vi "TCPtaskhandle.vi"(6 "心跳包":refnum<vi>, 9 "配置信息":refnum<vi>, 10 "状态信息":refnum<vi>, 11 "通信状态":refnum<vi>) -> ()   [LabVIEW 2016, in "数据传输系统-06.lvlib"]
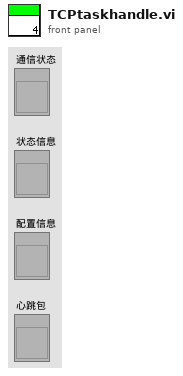
[diagram p1: front panel]
types:
  T1 = cluster{"步骤":enum16{"打开连接", "发送数据", "读取数据", "数据处理", "关闭连接"}, "发送报文":string}
  T2 = cluster{"setini":string, "sysini":string, "hechaini":string, "actualwrite":string, "actualread":string, "datasent":string, "反控命令信息队列":string, "反控与仪器交互":string}
  T3 = cluster{"1st Error to Convert ":i32, "步骤 ":enum16{"打开连接", "发送数据", "读取数据", "数据处理", "关闭连接"}, "元素":string, "TCP服务端掉线计数":i32, "TCP掉线时间节点":string}
  T4 = cluster{"站点":string, "设备":string, "IP":string, "PORT":string, "MN":string, "PW":string}
  T5 = cluster{"枚举":enum16{"打开连接", "发送数据", "读取数据", "数据处理", "关闭连接"}, "读取缓冲区":string}
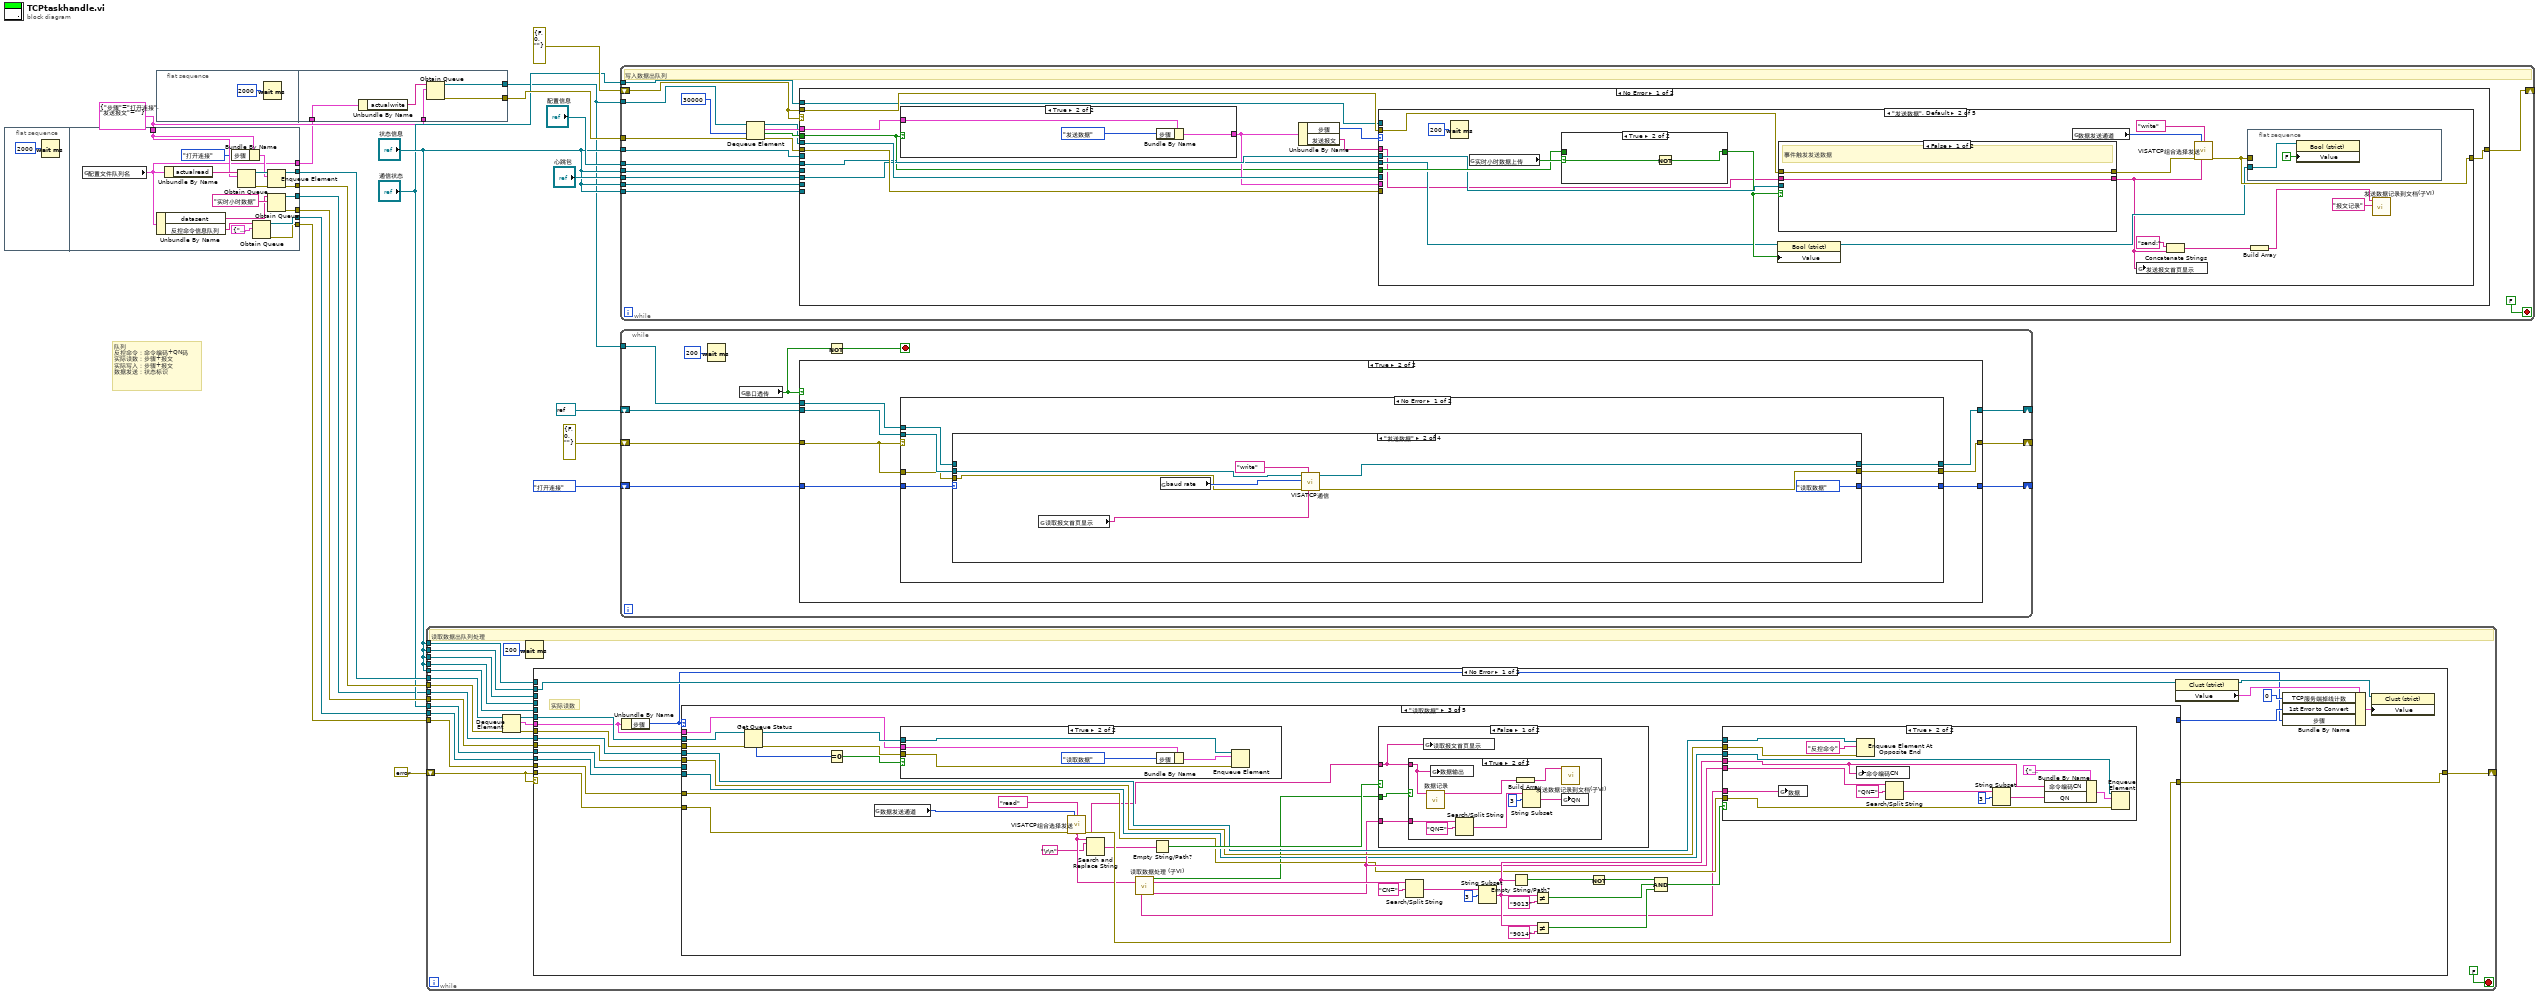
[diagram p0: block diagram]
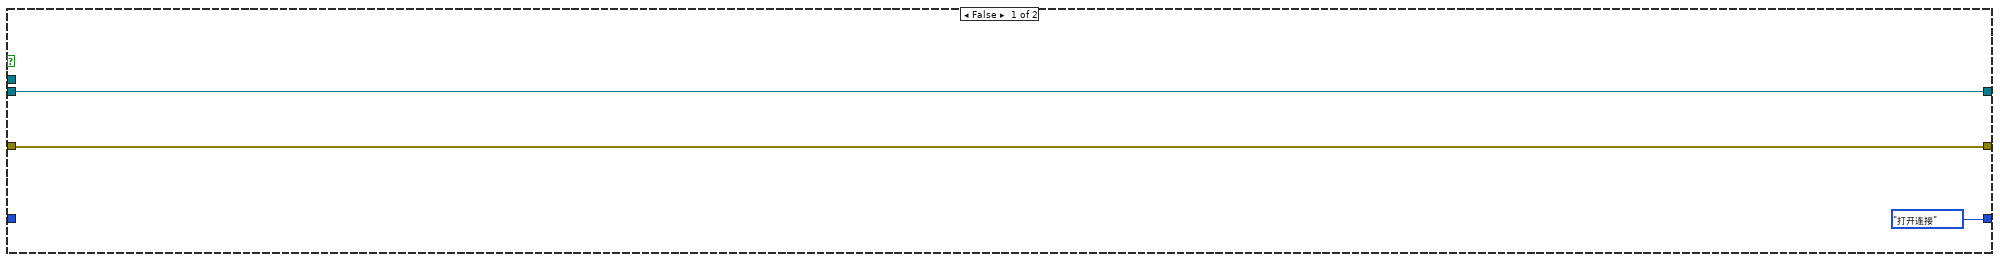
[diagram p2: hidden frame]
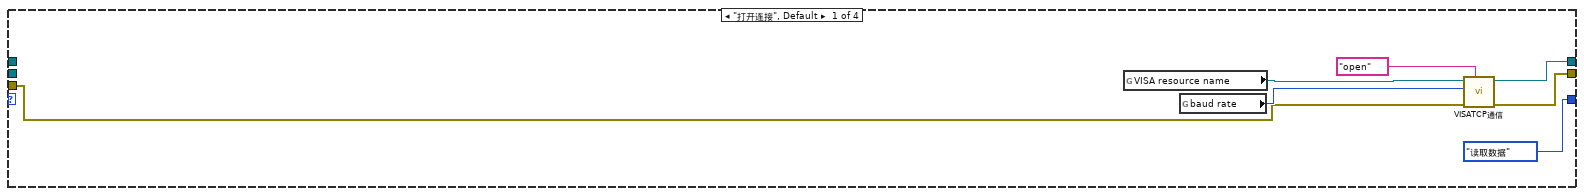
[diagram p3: hidden frame]
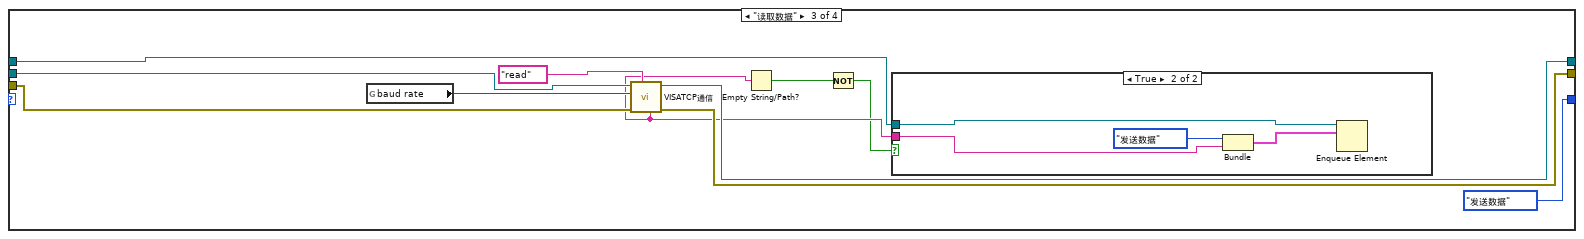
[diagram p4: hidden frame]
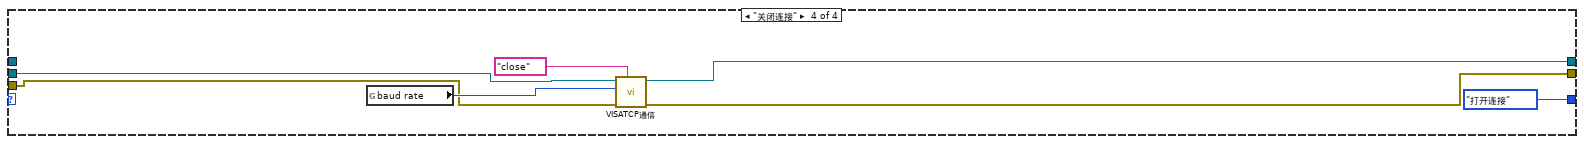
[diagram p6: hidden frame]
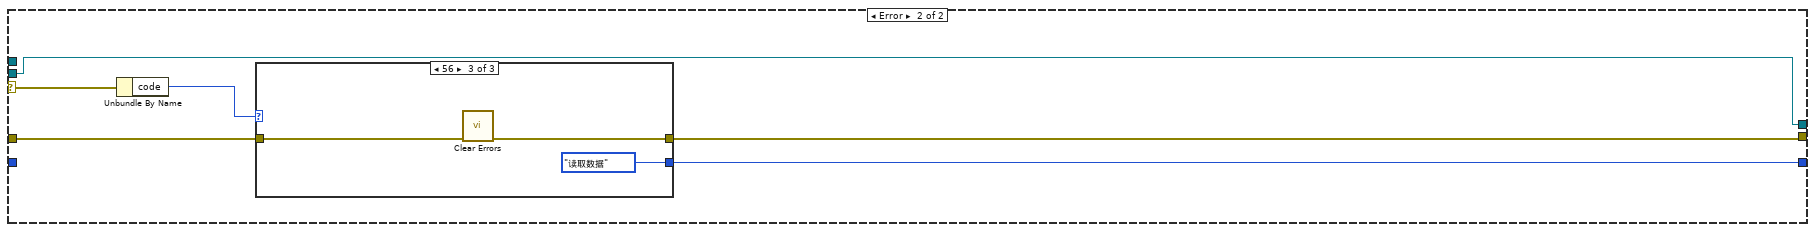
[diagram p7: hidden frame]
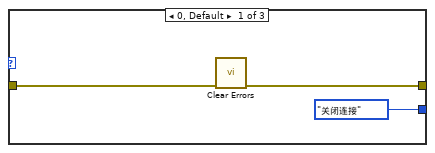
[diagram p8: hidden frame]
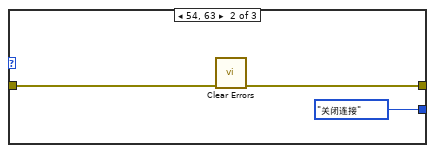
[diagram p9: hidden frame]
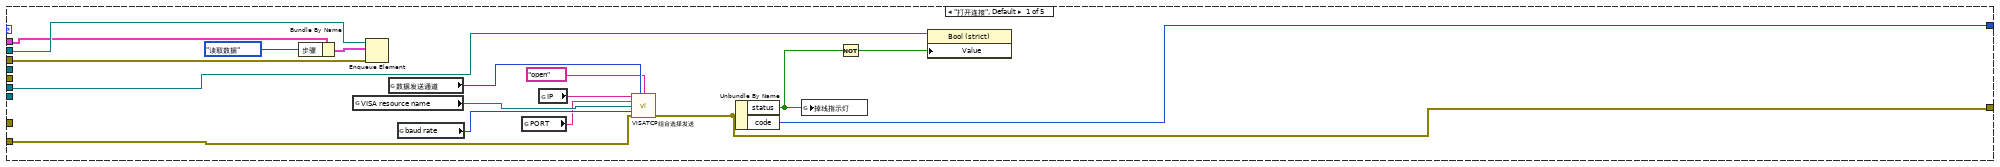
[diagram p10: hidden frame]
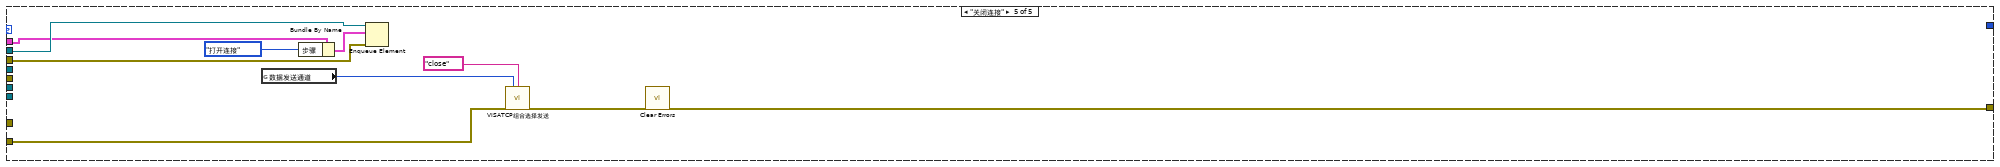
[diagram p17: hidden frame]
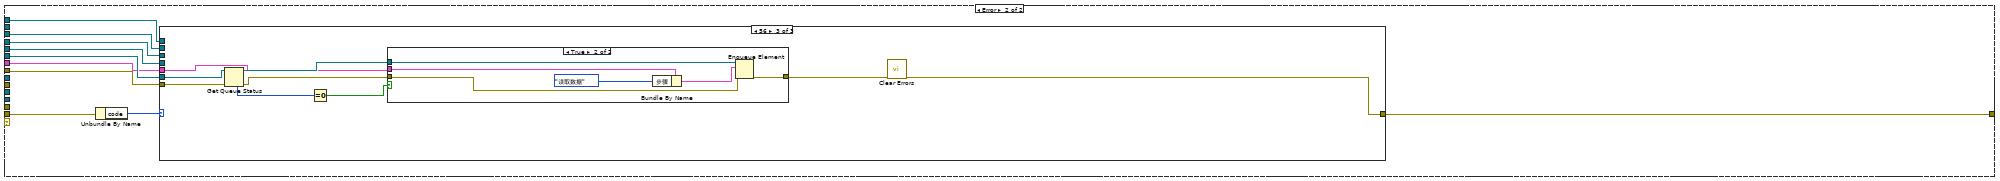
[diagram p18: hidden frame]
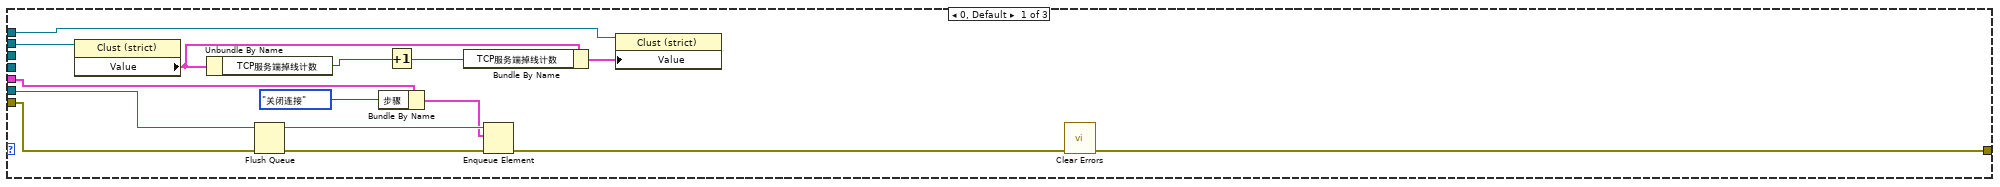
[diagram p19: hidden frame]
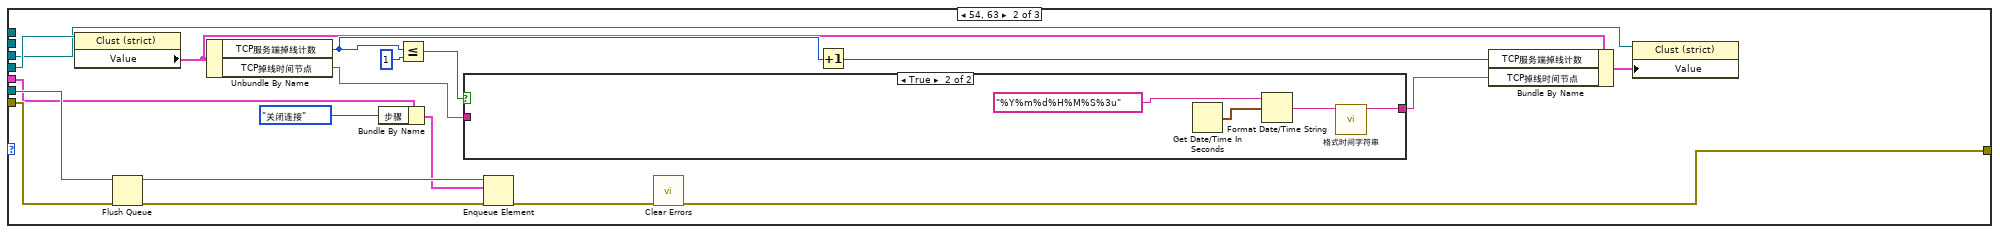
[diagram p20: hidden frame]
diagram:
  w7 = T1 {"步骤"=enum."打开连接", "发送报文"=""} ("data")
  # "队列\n反控命令：命令编码+QN码\n实际读数：步骤+报文\n实际写入：步骤+报文\n数据发送：状态标识"
  n1 = flat-sequence {
    tunnel: [w36] -> w14
    tunnel: [w35] -> w15
    tunnel: [w33] -> w1
    tunnel: [w32] -> w17
    tunnel: [w30] -> w18
    tunnel: [w29] -> w19
    tunnel: w7 -> [w24]
    tunnel: [w21] -> w6
    frame #0 {
      n2 = Wait (ms)(milliseconds to wait=u32 2000 ("等待时间（毫秒）")) -> ()  [unwired: 1 out]
    }
    frame #1 {
      n3 = global read "全局1.vi" "配置文件队列名"() -> (w21:T2)
      n4 = Unbundle By Name(w21) -> ("datasent"=w26:string, "反控命令信息队列"=w25:string)
      n5 = Unbundle By Name(w21) -> ("actualread"=w27:string)
      n6 = Bundle By Name(cluster=w24, "步骤"=enum16{"打开连接", "发送数据", "读取数据", "数据处理", "关闭连接"}."打开连接" ("枚举")) -> (w22:T1)
      n7 = Obtain Queue(name (unnamed)=w27, element data type=w24) -> (queue out=w37:refnum<queue>, error out=w34:errorcluster)  [unwired: 3 in, 1 out]
      n8 = Obtain Queue(name (unnamed)=w25, element data type=cluster{"命令编码CN":string, "QN":string} {"命令编码CN"="", "QN"=""}) -> (queue out=w30:refnum<queue>, error out=w29:errorcluster)  [unwired: 3 in, 1 out]
      n9 = Enqueue Element(queue=w37, element=w22, error in (no error)=w34) -> (queue out=w36:refnum<queue>, error out=w35:errorcluster)  [unwired: 1 in, 1 out]
      n10 = Obtain Queue(name (unnamed)=w26, element data type="实时小时数据" ("元素")) -> (queue out=w33:refnum<queue>, error out=w32:errorcluster)  [unwired: 3 in, 1 out]
    }
  }
  n11 = flat-sequence {
    tunnel: [w43] -> w2
    tunnel: [w42] -> w12
    tunnel: w7 -> [w40]
    tunnel: w6 -> [w39]
    frame #0 {
      n12 = Wait (ms)(milliseconds to wait=u32 2000 ("等待时间（毫秒）")) -> ()  [unwired: 1 out]
    }
    frame #1 {
      n13 = Unbundle By Name(w39) -> ("actualwrite"=w41:string)
      n14 = Obtain Queue(name (unnamed)=w41, element data type=w40) -> (queue out=w43:refnum<queue>, error out=w42:errorcluster)  [unwired: 3 in, 1 out]
    }
  }
  n15 = while {
    tunnel: w14 -> [w62]
    tunnel: w15 -> [w61]
    shift-right: [w58] -> _
    shift-left: errorcluster {"status"=FALSE, "code"=0, "source"=""} ("error out") -> [w57]
    tunnel: w1 -> [w53]
    tunnel: w17 -> [w52]
    tunnel: w18 -> [w51]
    tunnel: w19 -> [w50]
    tunnel: "状态信息" -> [w49]
    tunnel: "状态信息" -> [w48]
    tunnel: "状态信息" -> [w47]
    tunnel: "状态信息" -> [w46]
    tunnel: "状态信息" -> [w45]
    tunnel: "通信状态" -> [w44]
    stop <- FALSE stop-if-true
    # "读取数据出队列处理"
    n16 = Dequeue Element(queue=w62, error in (no error)=w61) -> (queue out=w56:refnum<queue>, element=w59:T1, error out=w55:errorcluster)  [unwired: 1 in, 1 out]
    n17 = Wait (ms)(milliseconds to wait=u32 200 ("等待时间（毫秒）")) -> ()  [unwired: 1 out]
    n18 = case shown="No Error" w57 {
      tunnel: w59 -> [w63 w171]
      tunnel: [w79 w176] -> w58
      tunnel: w57 -> [w78 w180]
      tunnel: w56 -> [w77 w178]
      tunnel: w55 -> [w76 w177]
      tunnel: w53 -> [w72 _]
      tunnel: w52 -> [w71 _]
      tunnel: w51 -> [w70 _]
      tunnel: w50 -> [w69 _]
      tunnel: w49 -> [w68 _]
      tunnel: w48 -> [_ w175]
      tunnel: w47 -> [_ w174]
      tunnel: w46 -> [_ w173]
      tunnel: w45 -> [_ w172]
      tunnel: w44 -> [w65 _]
      frame No Error {
        # "实际读数"
        n19 = Unbundle By Name(w63) -> ("步骤"=w64:enum16{"打开连接", "发送数据", "读取数据", "数据处理", "关闭连接"})
        n20 = case shown="\"读取数据\"" w64 {
          tunnel: [w90 _ w127 _ w166] -> w79
          tunnel: w78 -> [w89 _ w130 _ w167]
          tunnel: w77 -> [w88 _ w122 _ w165]
          tunnel: w76 -> [w87 _ w121 _ w164]
          tunnel: [w86 _ _ _ _] -> w74
          tunnel: w72 -> [_ _ w115 _ _]
          tunnel: w71 -> [_ _ w114 _ _]
          tunnel: w70 -> [_ _ w104 _ _]
          tunnel: w69 -> [_ _ w103 _ _]
          tunnel: w65 -> [w84 _ _ _ _]
          tunnel: w63 -> [w81 _ w102 _ w161]
          frame "打开连接", Default {
            n21 = Bundle By Name(cluster=w81, "步骤"=enum16{"打开连接", "发送数据", "读取数据", "数据处理", "关闭连接"}."读取数据" ("枚举")) -> (w80:T1)
            n22 = global read "断电保存全局.vi" "VISA resource name"() -> (w96:refnum<visa-resource-name>)
            n23 = Enqueue Element(queue=w88, element=w80, error in (no error)=w87) -> ()  [unwired: 1 in, 3 out]
            n24 = global read "断电保存全局.vi" "数据发送通道"() -> (w93:enum16{"TCP", "VISA"})
            n25 = global read "断电保存全局.vi" "baud rate"() -> (w95:u32)
            n26 = global read "断电保存全局.vi" "PORT"() -> (w94:string)
            n27 = global read "断电保存全局.vi" "IP"() -> (w92:string)
            n28 = call "VISATCP组合选择发送.vi"("IP"=w92, "数据发送通道"=w93, "命令"="open", "PORT"=w94, "VISA resource name"=w96, "baud rate"=w95, "error in (no error)"=w89) -> ("错误输出"=w90:errorcluster)  [unwired: 5 in, 3 out]
            n29 = Unbundle By Name(w90) -> ("status"=w85:bool, "code"=w86:i32)
            n30 = global write "全局 数据发送重叠.vi" "掉线指示灯"(w85) -> ()
            n31 = Not(x=w85) -> (.not. x?=w83:bool)
            n32 = property class="Bool (strict)"(reference=w84, "Value"=w83) -> ()  [unwired: 1 in, 2 out]
          }
          frame "发送数据" {
          }
          frame "读取数据" {
            n33 = Get Queue Status(queue=w122, error in (no error)=w121) -> (queue out=w118:refnum<queue>, error out=w117:errorcluster, # elements in queue=w120:i32)  [unwired: 1 in, 5 out]
            n34 = Equal To 0?(x=w120) -> (x = 0?=w119:bool)
            n35 = global read "断电保存全局.vi" "数据发送通道"() -> (w129:enum16{"TCP", "VISA"})
            n36 = case shown="True" w119 {
              tunnel: w118 -> [_ w160]
              tunnel: w117 -> [_ w159]
              tunnel: w102 -> [_ w158]
              frame False {
              }
              frame True {
                n37 = Bundle By Name(cluster=w158, "步骤"=enum16{"打开连接", "发送数据", "读取数据", "数据处理", "关闭连接"}."读取数据" ("枚举")) -> (w156:T1)
                n38 = Enqueue Element(queue=w160, element=w156, error in (no error)=w159) -> ()  [unwired: 1 in, 3 out]
              }
            }
            n39 = call "VISATCP组合选择发送.vi"("数据发送通道"=w129, "命令"="read", "error in (no error)"=w130) -> ("读取缓冲区"=w99:string, "错误输出"=w127:errorcluster)  [unwired: 9 in, 2 out]
            n40 = Search and Replace String(input string=w99, search string="\r\n") -> (result string=w100:string)  [unwired: 6 in, 3 out]
            n41 = call "读取数据处理 (子VI).vi"("data out"=w99) -> ("CHECK?"=w101:bool, "命令编码CN"=w123:string, "数据"=w97:string, "时间QN"=w105:string)  [unwired: 7 in, 4 out]
            n42 = Empty String/Path?(string/path=w100) -> (empty?=w116:bool)
            n43 = case shown="False" w116 {
              tunnel: w99 -> [w147 _]
              tunnel: w105 -> [w146 _]
              tunnel: w101 -> [w145 _]
              frame False {
                n44 = case shown="True" w145 {
                  tunnel: w147 -> [_ w153]
                  tunnel: w146 -> [_ w150]
                  frame False {
                  }
                  frame True {
                    n45 = call "数据记录.vi"("写入字段"=w153) -> ("连接的字符串"=w154:string)  [unwired: 10 in]
                    n46 = global write "全局1.vi" "数据输出"(w153) -> ()
                    n47 = Search/Split String(string=w150, search string/char (-)="QN=" ("搜索字符串/字符(-)")) -> (match + rest of string=w149:string)  [unwired: 1 in, 2 out]
                    n48 = Build Array(w154) -> (w155:string[])
                    n49 = String Subset(string=w149, offset (0)=3 ("偏移量(0)")) -> (substring=w148:string)  [unwired: 1 in]
                    n50 = call "发送数据记录到文档(子VI).vi"("数组"=w155) -> ()  [unwired: 9 in, 1 out]
                    n51 = global write "全局1.vi" "QN"(w148) -> ()
                  }
                }
                n52 = global write "全局1.vi" "读取报文首页显示"(w147) -> ()
              }
              frame True {
              }
            }
            n53 = Search/Split String(string=w123, search string/char (-)="CN=" ("搜索字符串/字符(-)")) -> (match + rest of string=w124:string)  [unwired: 1 in, 2 out]
            n54 = String Subset(string=w124, offset (0)=3 ("偏移量(0)")) -> (substring=w111:string)  [unwired: 1 in]
            n55 = Empty String/Path?(string/path=w111) -> (empty?=w113:bool)
            n56 = Not Equal?(x=w111, y="9013") -> (x != y?=w108:bool)
            n57 = Not Equal?(x=w111, y="9014") -> (x != y?=w107:bool)
            n58 = Not(x=w113) -> (.not. x?=w106:bool)
            n59 = Compound Arithmetic op=AND ("复合运算")(w106, w108, w107) -> (w112:bool)
            n60 = case shown="True" w112 {
              tunnel: w115 -> [_ w132]
              tunnel: w114 -> [_ w131]
              tunnel: w97 -> [_ w144]
              tunnel: w111 -> [_ w135]
              tunnel: w105 -> [_ w140]
              tunnel: w104 -> [_ w139]
              tunnel: w103 -> [_ w138]
              frame False {
              }
              frame True {
                n61 = global write "全局1.vi" "数据"(w144) -> ()
                n62 = Enqueue Element At Opposite End(queue=w132, element="反控命令" ("元素"), error in (no error)=w131) -> ()  [unwired: 1 in, 3 out]
                n63 = global write "全局1.vi" "命令编码CN"(w135) -> ()
                n64 = Search/Split String(string=w140, search string/char (-)="QN=" ("搜索字符串/字符(-)")) -> (match + rest of string=w143:string)  [unwired: 1 in, 2 out]
                n65 = String Subset(string=w143, offset (0)=3 ("偏移量(0)")) -> (substring=w134:string)  [unwired: 1 in]
                n66 = Bundle By Name(cluster=cluster{"命令编码CN":string, "QN":string} {"命令编码CN"="", "QN"=""}, "命令编码CN"=w135, "QN"=w134) -> (w136:cluster{"命令编码CN":string, "QN":string})
                n67 = Enqueue Element(queue=w139, element=w136, error in (no error)=w138) -> ()  [unwired: 1 in, 3 out]
              }
            }
          }
          frame "数据处理" {
          }
          frame "关闭连接" {
            n68 = global read "断电保存全局.vi" "数据发送通道"() -> (w169:enum16{"TCP", "VISA"})
            n69 = Bundle By Name(cluster=w161, "步骤"=enum16{"打开连接", "发送数据", "读取数据", "数据处理", "关闭连接"}."打开连接" ("枚举")) -> (w162:T1)
            n70 = Enqueue Element(queue=w165, element=w162, error in (no error)=w164) -> ()  [unwired: 1 in, 3 out]
            n71 = call "VISATCP组合选择发送.vi"("数据发送通道"=w169, "命令"="close", "error in (no error)"=w167) -> ("错误输出"=w168:errorcluster)  [unwired: 9 in, 3 out]
            n72 = call <vilib>:"Clear Errors.vi"("error in (no error)"=w168) -> ("error out"=w166:errorcluster)  [unwired: 5 in, 1 out]
          }
        }
        n73 = property class="Clust (strict)"(reference=w68) -> (reference out=w67:refnum<vi>, "Value"=w75:T3)  [unwired: 1 in, 1 out]
        n74 = Bundle By Name(cluster=w75, "TCP服务端掉线计数"=0, "1st Error to Convert"=w74, "步骤"=w64) -> (w66:T3)
        n75 = property class="Clust (strict)"(reference=w67, "Value"=w66) -> ()  [unwired: 1 in, 2 out]
      }
      frame Error {
        n76 = Unbundle By Name(w180) -> ("code"=w179:i32)
        n77 = case shown="56" w179 {
          tunnel: w178 -> [w192 w212 w222]
          tunnel: w177 -> [w191 w211 w221]
          tunnel: [w190 w209 w228] -> w176
          tunnel: w175 -> [w185 _ _]
          tunnel: w174 -> [w184 _ _]
          tunnel: w173 -> [_ w200 _]
          tunnel: w172 -> [_ w199 _]
          tunnel: w171 -> [w183 w198 w220]
          frame 0, Default {
            n78 = property class="Clust (strict)"(reference=w185) -> ("Value"=w189:T3)  [unwired: 1 in, 2 out]
            n79 = Unbundle By Name(w189) -> ("TCP服务端掉线计数"=w187:i32)
            n80 = Flush Queue(queue=w192, error in (no error)=w191) -> (queue out=w193:refnum<queue>, error out=w194:errorcluster)  [unwired: 1 out]
            n81 = Bundle By Name(cluster=w183, "步骤"=enum16{"打开连接", "发送数据", "读取数据", "数据处理", "关闭连接"}."关闭连接" ("枚举")) -> (w181:T1)
            n82 = Increment(x=w187) -> (x+1=w188:i32)
            n83 = Bundle By Name(cluster=w189, "TCP服务端掉线计数"=w188) -> (w186:T3)
            n84 = Enqueue Element(queue=w193, element=w181, error in (no error)=w194) -> (error out=w195:errorcluster)  [unwired: 1 in, 2 out]
            n85 = property class="Clust (strict)"(reference=w184, "Value"=w186) -> ()  [unwired: 1 in, 2 out]
            n86 = call <vilib>:"Clear Errors.vi"("error in (no error)"=w195) -> ("error out"=w190:errorcluster)  [unwired: 5 in, 1 out]
          }
          frame 54, 63 {
            n87 = property class="Clust (strict)"(reference=w200) -> ("Value"=w204:T3)  [unwired: 1 in, 2 out]
            n88 = Flush Queue(queue=w212, error in (no error)=w211) -> (queue out=w213:refnum<queue>, error out=w214:errorcluster)  [unwired: 1 out]
            n89 = Unbundle By Name(w204) -> ("TCP服务端掉线计数"=w208:i32, "TCP掉线时间节点"=w201:string)
            n90 = Bundle By Name(cluster=w198, "步骤"=enum16{"打开连接", "发送数据", "读取数据", "数据处理", "关闭连接"}."关闭连接" ("枚举")) -> (w196:T1)
            n91 = Less Or Equal?(x=w208, y=1) -> (x <= y?=w206:bool)
            n92 = case shown="True" w206 {
              tunnel: [w215 w216] -> w205
              tunnel: w201 -> [w215 _]
              frame False {
              }
              frame True {
                n93 = Get Date/Time In Seconds() -> (seconds since 1Jan1904=w217:timestamp)
                n94 = Format Date/Time String(time format string (%c)="%Y%m%d%H%M%S%3u" ("时间格式字符串(%c)"), seconds (now)=w217) -> (date/time string=w219:string)  [unwired: 1 in]
                n95 = call "格式时间字符串.vi"("字符串"=w219) -> ("连接的字符串"=w216:string)  [unwired: 10 in]
              }
            }
            n96 = Enqueue Element(queue=w213, element=w196, error in (no error)=w214) -> (error out=w210:errorcluster)  [unwired: 1 in, 2 out]
            n97 = call <vilib>:"Clear Errors.vi"("error in (no error)"=w210) -> ("error out"=w209:errorcluster)  [unwired: 5 in, 1 out]
            n98 = Increment(x=w208) -> (x+1=w203:i32)
            n99 = Bundle By Name(cluster=w204, "TCP服务端掉线计数"=w203, "TCP掉线时间节点"=w205) -> (w202:T3)
            n100 = property class="Clust (strict)"(reference=w199, "Value"=w202) -> ()  [unwired: 1 in, 2 out]
          }
          frame 56 {
            n101 = Get Queue Status(queue=w222, error in (no error)=w221) -> (queue out=w224:refnum<queue>, error out=w223:errorcluster, # elements in queue=w226:i32)  [unwired: 1 in, 5 out]
            n102 = Equal To 0?(x=w226) -> (x = 0?=w225:bool)
            n103 = case shown="True" w225 {
              tunnel: [w229 w235] -> w227
              tunnel: w224 -> [_ w234]
              tunnel: w223 -> [w229 w233]
              tunnel: w220 -> [_ w231]
              frame False {
              }
              frame True {
                n104 = Bundle By Name(cluster=w231, "步骤"=enum16{"打开连接", "发送数据", "读取数据", "数据处理", "关闭连接"}."读取数据" ("枚举")) -> (w230:T1)
                n105 = Enqueue Element(queue=w234, element=w230, error in (no error)=w233) -> (error out=w235:errorcluster)  [unwired: 1 in, 2 out]
              }
            }
            n106 = call <vilib>:"Clear Errors.vi"("error in (no error)"=w227) -> ("error out"=w228:errorcluster)  [unwired: 5 in, 1 out]
          }
        }
      }
    }
  }
  n107 = while {
    tunnel: w2 -> [w251]
    tunnel: w12 -> [w250]
    shift-right: [w246] -> _
    shift-left: errorcluster {"status"=FALSE, "code"=0, "source"=""} ("error out") -> [w245]
    tunnel: "通信状态" -> [w242]
    tunnel: "配置信息" -> [w241]
    tunnel: "心跳包" -> [w240]
    tunnel: "状态信息" -> [w239]
    tunnel: "状态信息" -> [w238]
    tunnel: "状态信息" -> [w237]
    tunnel: "状态信息" -> [w236]
    stop <- FALSE stop-if-true
    # "写入数据出队列"
    n108 = Dequeue Element(queue=w251, timeout in ms (-1)=30000 ("超时毫秒(-1)"), error in (no error)=w250) -> (queue out=w244:refnum<queue>, element=w248:T1, timed out?=w247:bool, error out=w243:errorcluster)
    n109 = case shown="No Error" w245 {
      tunnel: w248 -> [w260 w322]
      tunnel: w247 -> [w253 _]
      tunnel: [w264 w327] -> w246
      tunnel: w245 -> [w263 w331]
      tunnel: w244 -> [w262 w329]
      tunnel: w243 -> [w261 w328]
      tunnel: w242 -> [w259 _]
      tunnel: w241 -> [w258 _]
      tunnel: w240 -> [w254 _]
      tunnel: w239 -> [_ w326]
      tunnel: w238 -> [_ w325]
      tunnel: w237 -> [_ w324]
      tunnel: w236 -> [_ w323]
      frame No Error {
        n110 = case shown="True" w253 {
          tunnel: [w318 w319] -> w255
          tunnel: w260 -> [w318 w321]
          frame False {
          }
          frame True {
            n111 = Bundle By Name(cluster=w321, "步骤"=enum16{"打开连接", "发送数据", "读取数据", "数据处理", "关闭连接"}."发送数据" ("枚举")) -> (w319:T1)
          }
        }
        n112 = Unbundle By Name(w255) -> ("步骤"=w257:enum16{"打开连接", "发送数据", "读取数据", "数据处理", "关闭连接"}, "发送报文"=w256:string)
        n113 = case shown="\"发送数据\", Default" w257 {
          tunnel: w253 -> [_ w283 _ _ _]
          tunnel: [w267 w286 _ _ w312] -> w264
          tunnel: w263 -> [w269 w291 _ _ w313]
          tunnel: w262 -> [_ _ _ _ w314]
          tunnel: w261 -> [_ _ _ _ w311]
          tunnel: w259 -> [w265 _ _ _ _]
          tunnel: w258 -> [_ w282 _ _ _]
          tunnel: w254 -> [_ w280 _ _ _]
          tunnel: w256 -> [_ w278 _ _ _]
          tunnel: w255 -> [_ _ _ _ w309]
          frame "打开连接" {
            n114 = global read "断电保存全局.vi" "VISA resource name"() -> (w275:refnum<visa-resource-name>)
            n115 = global read "断电保存全局.vi" "数据发送通道"() -> (w272:enum16{"TCP", "VISA"})
            n116 = global read "断电保存全局.vi" "baud rate"() -> (w274:u32)
            n117 = global read "断电保存全局.vi" "PORT"() -> (w273:string)
            n118 = global read "断电保存全局.vi" "IP"() -> (w271:string)
            n119 = call "VISATCP组合选择发送.vi"("IP"=w271, "数据发送通道"=w272, "命令"="open", "PORT"=w273, "VISA resource name"=w275, "baud rate"=w274, "error in (no error)"=w269) -> ("错误输出"=w267:errorcluster)  [unwired: 5 in, 3 out]
            n120 = Unbundle By Name(w267) -> ("status"=w266:bool)  [unwired: 1 out]
            n121 = global write "全局 数据发送重叠.vi" "掉线指示灯"(w266) -> ()
            n122 = Not(x=w266) -> (.not. x?=w268:bool)
            n123 = property class="Bool (strict)"(reference=w265, "Value"=w268) -> ()  [unwired: 1 in, 2 out]
          }
          frame "发送数据", Default {
            n124 = Wait (ms)(milliseconds to wait=u32 200 ("等待时间（毫秒）")) -> ()  [unwired: 1 out]
            n125 = global read "全局1.vi" "实时小时数据上传"() -> (w284:bool)
            n126 = case shown="True" w284 {
              selector: w284 -> [_ w307]
              tunnel: w283 -> [w305 _]
              tunnel: [w305 w306] -> w281
              frame False {
              }
              frame True {
                n127 = Not(x=w307) -> (.not. x?=w306:bool)
              }
            }
            n128 = property class="Bool (strict)"(reference=w280, "Value"=w281) -> (reference out=w279:refnum<vi>)  [unwired: 1 in, 1 out]
            n129 = case shown="False" w281 {
              tunnel: [w296 w299] -> w277
              tunnel: w291 -> [w297 w300]
              tunnel: [w297 w300] -> w290
              tunnel: w282 -> [_ w298]
              tunnel: w278 -> [w296 _]
              frame False {
                # "事件触发发送数据"
              }
              frame True {
                # "30秒超时发送心跳包"
                n130 = property class="Clust (strict)"(reference=w298) -> ("Value"=w303:T4)  [unwired: 1 in, 2 out]
                n131 = Unbundle By Name(w303) -> ("MN"=w302:string, "PW"=w301:string)
                n132 = call "数据编码.vi"("table输入"="心跳包", "MN"=w302, "PW"=w301) -> ("通讯包字符串"=w299:string)  [unwired: 11 in, 1 out]
              }
            }
            n133 = global read "断电保存全局.vi" "数据发送通道"() -> (w292:enum16{"TCP", "VISA"})
            n134 = global write "全局1.vi" "发送报文首页显示"(w277) -> ()
            n135 = Concatenate Strings("send:" ("字符串"), w277) -> (w287:string)
            n136 = call "VISATCP组合选择发送.vi"("数据发送通道"=w292, "命令"="write", "error in (no error)"=w290, "写入缓冲区"=w277) -> ("错误输出"=w286:errorcluster)  [unwired: 8 in, 3 out]
            n137 = flat-sequence {
              tunnel: w286 -> [_]
              tunnel: w279 -> [w294]
              frame #0 {
                n138 = property class="Bool (strict)"(reference=w294, "Value"=FALSE ("心跳包")) -> ()  [unwired: 1 in, 2 out]
              }
            }
            n139 = Build Array(w287) -> (w289:string[])
            n140 = call "发送数据记录到文档(子VI).vi"("字符串"="报文记录", "数组"=w289) -> ()  [unwired: 8 in, 1 out]
          }
          frame "读取数据" {
          }
          frame "数据处理" {
          }
          frame "关闭连接" {
            n141 = global read "断电保存全局.vi" "数据发送通道"() -> (w316:enum16{"TCP", "VISA"})
            n142 = Bundle By Name(cluster=w309, "步骤"=enum16{"打开连接", "发送数据", "读取数据", "数据处理", "关闭连接"}."打开连接" ("枚举")) -> (w308:T1)
            n143 = Enqueue Element(queue=w314, element=w308, error in (no error)=w311) -> ()  [unwired: 1 in, 3 out]
            n144 = call "VISATCP组合选择发送.vi"("数据发送通道"=w316, "命令"="write", "error in (no error)"=w313) -> ("错误输出"=w317:errorcluster)  [unwired: 9 in, 3 out]
            n145 = call <vilib>:"Clear Errors.vi"("error in (no error)"=w317) -> ("error out"=w312:errorcluster)  [unwired: 5 in, 1 out]
          }
        }
      }
      frame Error {
        n146 = Unbundle By Name(w331) -> ("code"=w330:i32)
        n147 = case shown="0, Default" w330 {
          tunnel: w329 -> [w343 w363 w374]
          tunnel: w328 -> [w342 w362 w373]
          tunnel: [w341 w360 w372] -> w327
          tunnel: w326 -> [w336 _ _]
          tunnel: w325 -> [w335 _ _]
          tunnel: w324 -> [_ w351 _]
          tunnel: w323 -> [_ w350 _]
          tunnel: w322 -> [w333 w349 _]
          frame 0, Default {
            n148 = property class="Clust (strict)"(reference=w336) -> ("Value"=w340:T3)  [unwired: 1 in, 2 out]
            n149 = Unbundle By Name(w340) -> ("TCP服务端掉线计数"=w338:i32)
            n150 = Flush Queue(queue=w343, error in (no error)=w342) -> (queue out=w344:refnum<queue>, error out=w345:errorcluster)  [unwired: 1 out]
            n151 = Bundle By Name(cluster=w333, "步骤"=enum16{"打开连接", "发送数据", "读取数据", "数据处理", "关闭连接"}."关闭连接" ("枚举")) -> (w332:T1)
            n152 = Increment(x=w338) -> (x+1=w339:i32)
            n153 = Bundle By Name(cluster=w340, "TCP服务端掉线计数"=w339) -> (w337:T3)
            n154 = Enqueue Element(queue=w344, element=w332, error in (no error)=w345) -> (error out=w346:errorcluster)  [unwired: 1 in, 2 out]
            n155 = property class="Clust (strict)"(reference=w335, "Value"=w337) -> ()  [unwired: 1 in, 2 out]
            n156 = call <vilib>:"Clear Errors.vi"("error in (no error)"=w346) -> ("error out"=w341:errorcluster)  [unwired: 5 in, 1 out]
          }
          frame 54, 63 {
            n157 = property class="Clust (strict)"(reference=w351) -> ("Value"=w355:T3)  [unwired: 1 in, 2 out]
            n158 = Flush Queue(queue=w363, error in (no error)=w362) -> (queue out=w364:refnum<queue>, error out=w365:errorcluster)  [unwired: 1 out]
            n159 = Unbundle By Name(w355) -> ("TCP服务端掉线计数"=w359:i32, "TCP掉线时间节点"=w352:string)
            n160 = Bundle By Name(cluster=w349, "步骤"=enum16{"打开连接", "发送数据", "读取数据", "数据处理", "关闭连接"}."关闭连接" ("枚举")) -> (w347:T1)
            n161 = Less Or Equal?(x=w359, y=1) -> (x <= y?=w357:bool)
            n162 = case shown="True" w357 {
              tunnel: [w366 w367] -> w356
              tunnel: w352 -> [w366 _]
              frame False {
              }
              frame True {
                n163 = Get Date/Time In Seconds() -> (seconds since 1Jan1904=w368:timestamp)
                n164 = Format Date/Time String(time format string (%c)="%Y%m%d%H%M%S%3u" ("时间格式字符串(%c)"), seconds (now)=w368) -> (date/time string=w370:string)  [unwired: 1 in]
                n165 = call "格式时间字符串.vi"("字符串"=w370) -> ("连接的字符串"=w367:string)  [unwired: 10 in]
              }
            }
            n166 = Enqueue Element(queue=w364, element=w347, error in (no error)=w365) -> (error out=w361:errorcluster)  [unwired: 1 in, 2 out]
            n167 = call <vilib>:"Clear Errors.vi"("error in (no error)"=w361) -> ("error out"=w360:errorcluster)  [unwired: 5 in, 1 out]
            n168 = Increment(x=w359) -> (x+1=w354:i32)
            n169 = Bundle By Name(cluster=w355, "TCP服务端掉线计数"=w354, "TCP掉线时间节点"=w356) -> (w353:T3)
            n170 = property class="Clust (strict)"(reference=w350, "Value"=w353) -> ()  [unwired: 1 in, 2 out]
          }
          frame 56 {
            n171 = Flush Queue(queue=w374, error in (no error)=w373) -> (error out=w371:errorcluster)  [unwired: 2 out]
            n172 = call <vilib>:"Clear Errors.vi"("error in (no error)"=w371) -> ("error out"=w372:errorcluster)  [unwired: 5 in, 1 out]
          }
        }
      }
    }
  }
  n173 = while {
    shift-right: [w383] -> _
    shift-left: enum16{"打开连接", "发送数据", "读取数据", "数据处理", "关闭连接"}."打开连接" ("枚举") -> [w384]
    shift-right: [w379] -> _
    shift-left: refnum<visa-resource-name> refnum ("VISA resource name 2") -> [w378]
    shift-right: [w377] -> _
    shift-left: errorcluster {"status"=FALSE, "code"=0, "source"=""} ("错误输出") -> [w376]
    tunnel: w2 -> [w375]
    stop <- w380 stop-if-true
    n174 = Wait (ms)(milliseconds to wait=u32 200 ("等待时间（毫秒）")) -> ()  [unwired: 1 out]
    n175 = global read "断电保存全局.vi" "串口透传"() -> (w381:bool)
    n176 = case shown="True" w381 {
      tunnel: w384 -> [_ w394]
      tunnel: [enum16{"打开连接", "发送数据", "读取数据", "数据处理", "关闭连接"}."打开连接" ("枚举") w390] -> w383
      tunnel: [w386 w393] -> w379
      tunnel: w378 -> [w386 w392]
      tunnel: [w385 w391] -> w377
      tunnel: w376 -> [w385 w389]
      tunnel: w375 -> [_ w388]
      frame False {
      }
      frame True {
        n177 = case shown="No Error" w389 {
          selector: w389 -> [_ w443]
          tunnel: w394 -> [w401 _]
          tunnel: [w400 w444] -> w393
          tunnel: w392 -> [w399 w444]
          tunnel: [w398 w440] -> w391
          tunnel: w389 -> [w397 w441]
          tunnel: [w396 w439] -> w390
          tunnel: w388 -> [w395 _]
          frame No Error {
            n178 = case shown="\"发送数据\"" w401 {
              tunnel: [w405 w411 w424 w434] -> w400
              tunnel: w399 -> [_ w414 w426 w436]
              tunnel: [w404 w412 w423 w433] -> w398
              tunnel: w397 -> [w403 w413 w422 w435]
              tunnel: [enum16{"打开连接", "发送数据", "读取数据", "数据处理", "关闭连接"}."读取数据" ("枚举") enum16{"打开连接", "发送数据", "读取数据", "数据处理", "关闭连接"}."读取数据" ("枚举") enum16{"打开连接", "发送数据", "读取数据", "数据处理", "关闭连接"}."发送数据" ("枚举") enum16{"打开连接", "发送数据", "读取数据", "数据处理", "关闭连接"}."打开连接" ("枚举")] -> w396
              tunnel: w395 -> [_ _ w417 _]
              frame "打开连接", Default {
                n179 = global read "断电保存全局.vi" "VISA resource name"() -> (w407:refnum<visa-resource-name>)
                n180 = global read "断电保存全局.vi" "baud rate"() -> (w406:u32)
                n181 = call-poly "VISATCP通信.vi"("命令"="open", "error in (no error)"=w403, "baud rate (9600)"=w406, "VISA resource name"=w407) -> ("错误输出"=w404:errorcluster, "VISA resource name 2"=w405:refnum<visa-resource-name>)  [unwired: 5 in, 1 out]
              }
              frame "发送数据" {
                n182 = global read "全局1.vi" "读取报文首页显示"() -> (w409:string)
                n183 = global read "断电保存全局.vi" "baud rate"() -> (w415:u32)
                n184 = call-poly "VISATCP通信.vi"("写入缓冲区"=w409, "命令"="write", "error in (no error)"=w413, "baud rate (9600)"=w415, "VISA resource name"=w414) -> ("错误输出"=w412:errorcluster, "VISA resource name 2"=w411:refnum<visa-resource-name>)  [unwired: 4 in, 1 out]
              }
              frame "读取数据" {
                n185 = global read "断电保存全局.vi" "baud rate"() -> (w425:u32)
                n186 = call-poly "VISATCP通信.vi"("命令"="read", "error in (no error)"=w422, "baud rate (9600)"=w425, "VISA resource name"=w426) -> ("错误输出"=w423:errorcluster, "VISA resource name 2"=w424:refnum<visa-resource-name>, "读取缓冲区"=w419:string)  [unwired: 5 in]
                n187 = Empty String/Path?(string/path=w419) -> (empty?=w420:bool)
                n188 = Not(x=w420) -> (.not. x?=w418:bool)
                n189 = case shown="True" w418 {
                  tunnel: w419 -> [_ w430]
                  tunnel: w417 -> [_ w428]
                  frame False {
                  }
                  frame True {
                    n190 = Bundle("枚举"=enum16{"打开连接", "发送数据", "读取数据", "数据处理", "关闭连接"}."发送数据", "读取缓冲区"=w430) -> (w431:T5)  [unwired: 1 in]
                    n191 = Enqueue Element(queue=w428, element=w431) -> ()  [unwired: 2 in, 3 out]
                  }
                }
              }
              frame "关闭连接" {
                n192 = global read "断电保存全局.vi" "baud rate"() -> (w437:u32)
                n193 = call-poly "VISATCP通信.vi"("命令"="close", "error in (no error)"=w435, "baud rate (9600)"=w437, "VISA resource name"=w436) -> ("错误输出"=w433:errorcluster, "VISA resource name 2"=w434:refnum<visa-resource-name>)  [unwired: 5 in, 1 out]
              }
            }
          }
          frame Error {
            n194 = Unbundle By Name(w443) -> ("code"=w442:i32)
            n195 = case shown="56" w442 {
              tunnel: w441 -> [w447 w448 w453]
              tunnel: [w446 w449 w452] -> w440
              tunnel: [enum16{"打开连接", "发送数据", "读取数据", "数据处理", "关闭连接"}."关闭连接" ("枚举") enum16{"打开连接", "发送数据", "读取数据", "数据处理", "关闭连接"}."关闭连接" ("枚举") enum16{"打开连接", "发送数据", "读取数据", "数据处理", "关闭连接"}."读取数据" ("枚举")] -> w439
              frame 0, Default {
                n196 = call <vilib>:"Clear Errors.vi"("error in (no error)"=w447) -> ("error out"=w446:errorcluster)  [unwired: 5 in, 1 out]
              }
              frame 54, 63 {
                n197 = call <vilib>:"Clear Errors.vi"("error in (no error)"=w448) -> ("error out"=w449:errorcluster)  [unwired: 5 in, 1 out]
              }
              frame 56 {
                n198 = call <vilib>:"Clear Errors.vi"("error in (no error)"=w453) -> ("error out"=w452:errorcluster)  [unwired: 5 in, 1 out]
              }
            }
          }
        }
      }
    }
    n199 = Not(x=w381) -> (.not. x?=w380:bool)
  }
